vi "2019-05-09_Challenges.vi"() -> ()   [LabVIEW 2018]
panel:
  out "불리언 3":bool
  in  "불리언 4":bool
  in  "불리언 2":bool
  out "눌린 횟수":i32
  out "웨이브폼 차트":i8[](graph)
  out "홀수":dbl[](array[numeric])
  out "짝수":dbl[](array[numeric])
  in  "배열":dbl[](array[numeric])
  in  "열거형":enum16{"1번", "2번", "3번", "4번"}(ring)
  in  "불리언":bool
  out "순환 횟수":dbl
  out "랜덤 숫자":i8
  in  "입력":i8
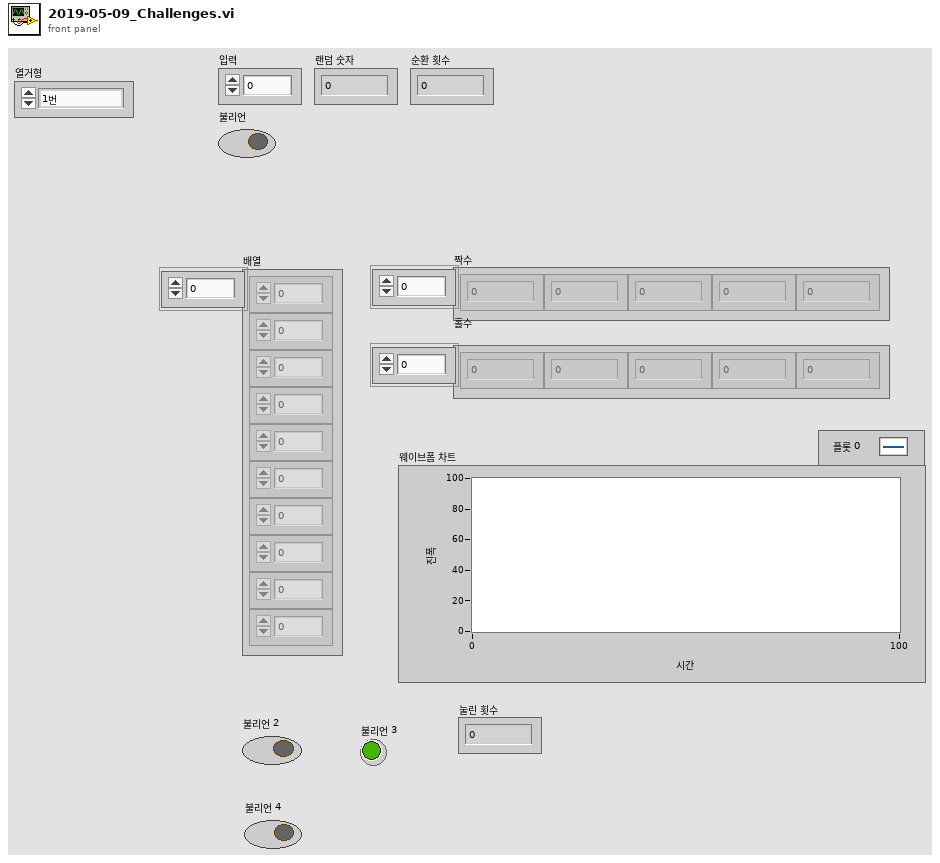
[diagram p1: front panel]
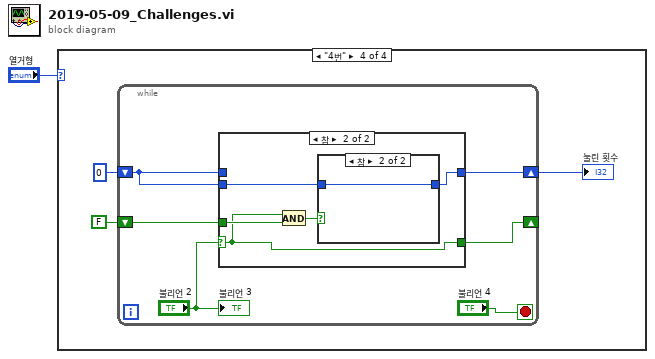
[diagram p0: block diagram]
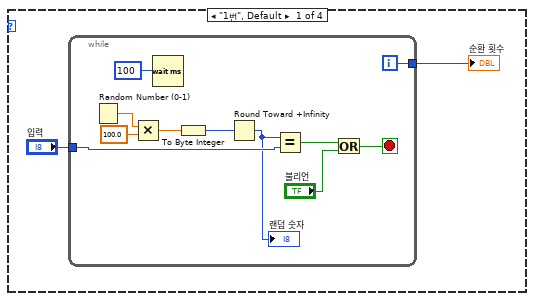
[diagram p2: hidden frame]
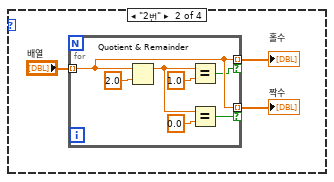
[diagram p3: hidden frame]
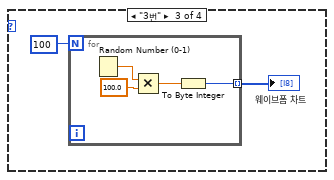
[diagram p4: hidden frame]
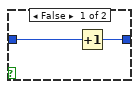
[diagram p6: hidden frame]
diagram:
  n1 = case shown="\"4번\"" "열거형" {
    frame "1번", Default {
      n2 = while {
        tunnel: "입력" -> [w10]
        tunnel: [w7] -> w3
        i -> [w7]
        stop <- w4 stop-if-true
        n3 = Random Number (0-1)() -> (number: 0 to 1=w14:dbl)
        n4 = Multiply(x=w14, y=100.0) -> (x*y=w12:dbl)
        n5 = Wait (ms)(milliseconds to wait=u32 100 ("대기 시간 (ms)")) -> ()  [unwired: 1 out]
        n6 = To Byte Integer(number=w12) -> (8bit integer=w11:i8)
        n7 = Round Toward +Infinity(x=w11) -> (ceil(x): smallest int >= x=w9:i8)
        "랜덤 숫자" <- w9
        n8 = Equal?(x=w9, y=w10) -> (x = y?=w6:bool)
        n9 = Or(x=w6, y="불리언") -> (x .or. y?=w4:bool)
      }
      "순환 횟수" <- w3
    }
    frame "2번" {
      n10 = for {
        tunnel: "배열" -> [w21] mode=indexing
        tunnel: [w21] -> w16 mode=indexing if=w22
        tunnel: [w21] -> w15 mode=indexing if=w18
        n11 = Quotient & Remainder(x=w21, y=2.0) -> (x-y*floor(x/y)=w19:dbl)  [unwired: 1 out]
        n12 = Equal?(x=w19, y=1.0) -> (x = y?=w18:bool)
        n13 = Equal?(x=w19, y=0.0) -> (x = y?=w22:bool)
      }
      "짝수" <- w16
      "홀수" <- w15
    }
    frame "3번" {
      n14 = for {
        N: 100 -> [_]
        tunnel: [w27] -> w25 mode=indexing
        n15 = Random Number (0-1)() -> (number: 0 to 1=w30:dbl)
        n16 = Multiply(x=w30, y=100.0) -> (x*y=w28:dbl)
        n17 = To Byte Integer(number=w28) -> (8bit integer=w27:i8)
      }
      "웨이브폼 차트" <- w25
    }
    frame "4번" {
      n18 = while {
        shift-right: [w38] -> w33
        shift-left: 0 -> [w34]
        shift-right: [w36] -> _
        shift-left: FALSE -> [w35]
        stop <- "불리언 4" stop-if-true
        n19 = case shown="참" "불리언 2" {
          selector: "불리언 2" -> [w40 w42]
          tunnel: [w41 w43] -> w38
          tunnel: w34 -> [w41 _]
          tunnel: [w40 w42] -> w36
          tunnel: w35 -> [_ w46]
          tunnel: w34 -> [_ w44]
          frame False {
          }
          frame True {
            n20 = And(x=w42, y=w46) -> (x .and. y?=w45:bool)
            n21 = case shown="참" w45 {
              tunnel: w44 -> [w48 w49]
              tunnel: [w47 w49] -> w43
              frame False {
                n22 = Increment(x=w48) -> (x+1=w47:i32)
              }
              frame True {
              }
            }
          }
        }
        "불리언 3" <- "불리언 2"
      }
      "눌린 횟수" <- w33
    }
  }
